vi "Target3.vi"() -> ()   [LabVIEW 2025]
uses:
  <vilib>/Platform/TimedLoop/XDataNode/timing_clust.ctl
  <vilib>/Platform/TimedLoop/XDataNode/nitl_modes.ctl
  <vilib>/Platform/TimedLoop/XDataNode/wakeup.ctl
  <vilib>/eio/utilities/niEioResolveVilibRelativePath.vi
  <vilib>/rvi/interface/RandomDataEmulation/niFpgaRandomDataHandleErrors.vi
  <vilib>/rvi/Emulation/niFpgaSctlEmulationGetInTimedLoop.vi
  <vilib>/rvi/Emulation/niFpgaEmulationReportErrorSimple.vi
  <vilib>/rvi/Emulation/niFpgaGetClockAttributes.vi
  <vilib>/rvi/Emulation/niFpgaCriticalErrorInLSC.vi
  <vilib>/rvi/linearAlgebra/MatrixMultiply/simVIs/SubVI/nifxpla_MatrixMultiply_SimMatrixSizes.vi
  <vilib>/rvi/linearAlgebra/MatrixMultiply/simVIs/SubVI/nifxpla_MatrixMultiply_Sim4WireAdapterVector.vi
  <vilib>/rvi/linearAlgebra/MatrixMultiply/simVIs/SubVI/nifxpla_MatrixMultiply_SimFrameHandShake.vi
  <vilib>/rvi/linearAlgebra/MatrixMultiply/simVIs/SubVI/nifxpla_MatrixMultiply_SimEndlessCounter.vi
  <vilib>/rvi/linearAlgebra/MatrixMultiply/simVIs/SubVI/nifxpla_MatrixMultiply_SimVectorDataBuffer.vi
  <vilib>/rvi/ClientSDK/Core/DevComputerLib/Private/Multiply(dfxp64).vi
  <vilib>/rvi/ClientSDK/Core/DevComputerLib/Private/Dfxp128ToDfxp256.vi
  <vilib>/rvi/ClientSDK/Core/DevComputerLib/Private/Add(dfxp256).vi
  <vilib>/rvi/ClientSDK/Core/DevComputerLib/Private/Subtract(dfxp256).vi
  <vilib>/rvi/ClientSDK/Core/DevComputerLib/Private/ToDfxp64(dfxp256).vi
  <vilib>/rvi/interface/RandomDataEmulation/nirviRandomDataMultiElementFPGAFIFO.vi
  <instcachedir>/0/nirviRandomDataMultiElementFPGAFIFO_BE2FF10D3D6E420AB0291A02835C249E.lvgen/nirviRandomDataMultiElementFPGAFIFO_BE2FF10D3D6E420AB0291A02835C249E_001.vi
  <vilib>/rvi/DataTransferAndStorage/Container/XNode/niFpgaContainer.xnode
  <vilib>/rvi/interface/RandomDataEmulation/nirviRandomDataFpgaReadWriteTemplate.vi
  <vilib>/platform/TimedLoop/XDataNode/XDataNode.xnode
  <vilib>/rvi/linearAlgebra/MatrixMultiply/XNode/nifxpla_MatrixMultiply.xnode
  <vilib>/rvi/linearAlgebra/MatrixMultiply/simVIs/nifxpla_MatrixMultiply_SimTemplateEinEout.vi
  <vilib>/rvi/linearAlgebra/MatrixMultiply/simVIs/nifxpla_MatrixMultiply_SimTemplateEinVout.vi
  <vilib>/rvi/linearAlgebra/MatrixMultiply/simVIs/nifxpla_MatrixMultiply_SimTemplateVinEout.vi
  <vilib>/rvi/linearAlgebra/MatrixMultiply/simVIs/nifxpla_MatrixMultiply_SimTemplateVinVout.vi
  <vilib>/rvi/interface/RandomDataEmulation/nirviRandomDataFpgaMultiElementTemplate.vi
  <vilib>/Platform/TimedLoop/XDataNode/XDNodeRunTimeDep.lvlib
panel:
  out "=0?2":bool
  out "=0?1":bool
  out "ready for b":bool[](array[boolean])
  out "ready for a":bool[](array[boolean])
  out "And 1":bool[](array[boolean])
  out "And 2":bool[](array[boolean])
  out "element 2":fxp<+/-,32,16>
  out "element":fxp<+/-,32,16>
  out "cr":fxp<+/-,32,16>[](array[numeric])
  out "Numeric 2":i32
  out "Array 3":fxp<+/-,32,16>[](array[numeric])
  out "Numeric":i32
  out "appended array 2":fxp<+/-,32,16>[](array[numeric])
  out "appended array":fxp<+/-,32,16>[](array[numeric])
  out "Ready for Input":bool
  out "output valid":bool
  out "operation overflow":bool
  out "Array 4":fxp<+/-,32,16>[](array[numeric])
  out "Array 5":fxp<+/-,32,16>[](array[numeric])
  out "Array 2":bool[](array[boolean])
  out "Array":bool[](array[boolean])
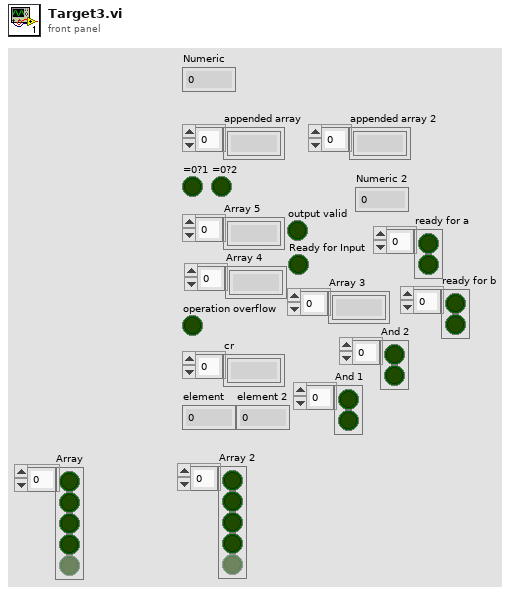
[diagram p1: front panel]
types:
  T1 = typedef "XDNodeRunTimeDep.lvlib/timing_clust.ctl" = cluster{"Expected End [f-1]":u64, "Actual End [f-1]":u64, "Finished Late? [f-1]":bool, "Expected End [i-1]":u64, "Actual End [i-1]":u64, "Finished Late? [i-1]":bool, "Expected Start [i]":u64, "Actual Start [i]":u64, "Expected Start [f]":u64, "Actual Start [f]":u64, "Source Name":string, "Structure Name":string, "Period":i64, "Deadline":i64, "Offset":i64, "Start":i64, "Priority":i32, "Timeout":i32, "Mode":T2, "Wakeup Reason":T3, "Error":errorcluster, "Source Type":string, "Secondary Source Type":string, "Global End Time":u64, "Global Start Time":u64, "Frame Duration":u64, "Iteration Duration":u64, "Assigned CPU":i32, "I/O Scan Engine Mode":u32}
  T2 = typedef "XDNodeRunTimeDep.lvlib/nitl_modes.ctl" = enum32{"No Change", "Process missed periods, maintain original phase", "Discard missed periods, maintain original phase", "Process missed periods, ignore original phase", "Discard missed periods, ignore original phase"}
  T3 = typedef "XDNodeRunTimeDep.lvlib/wakeup.ctl" = enum32{"Normal", "Aborted", "Asynchronous wakeup", "Timing source error", "Timed loop error", "Timeout"}
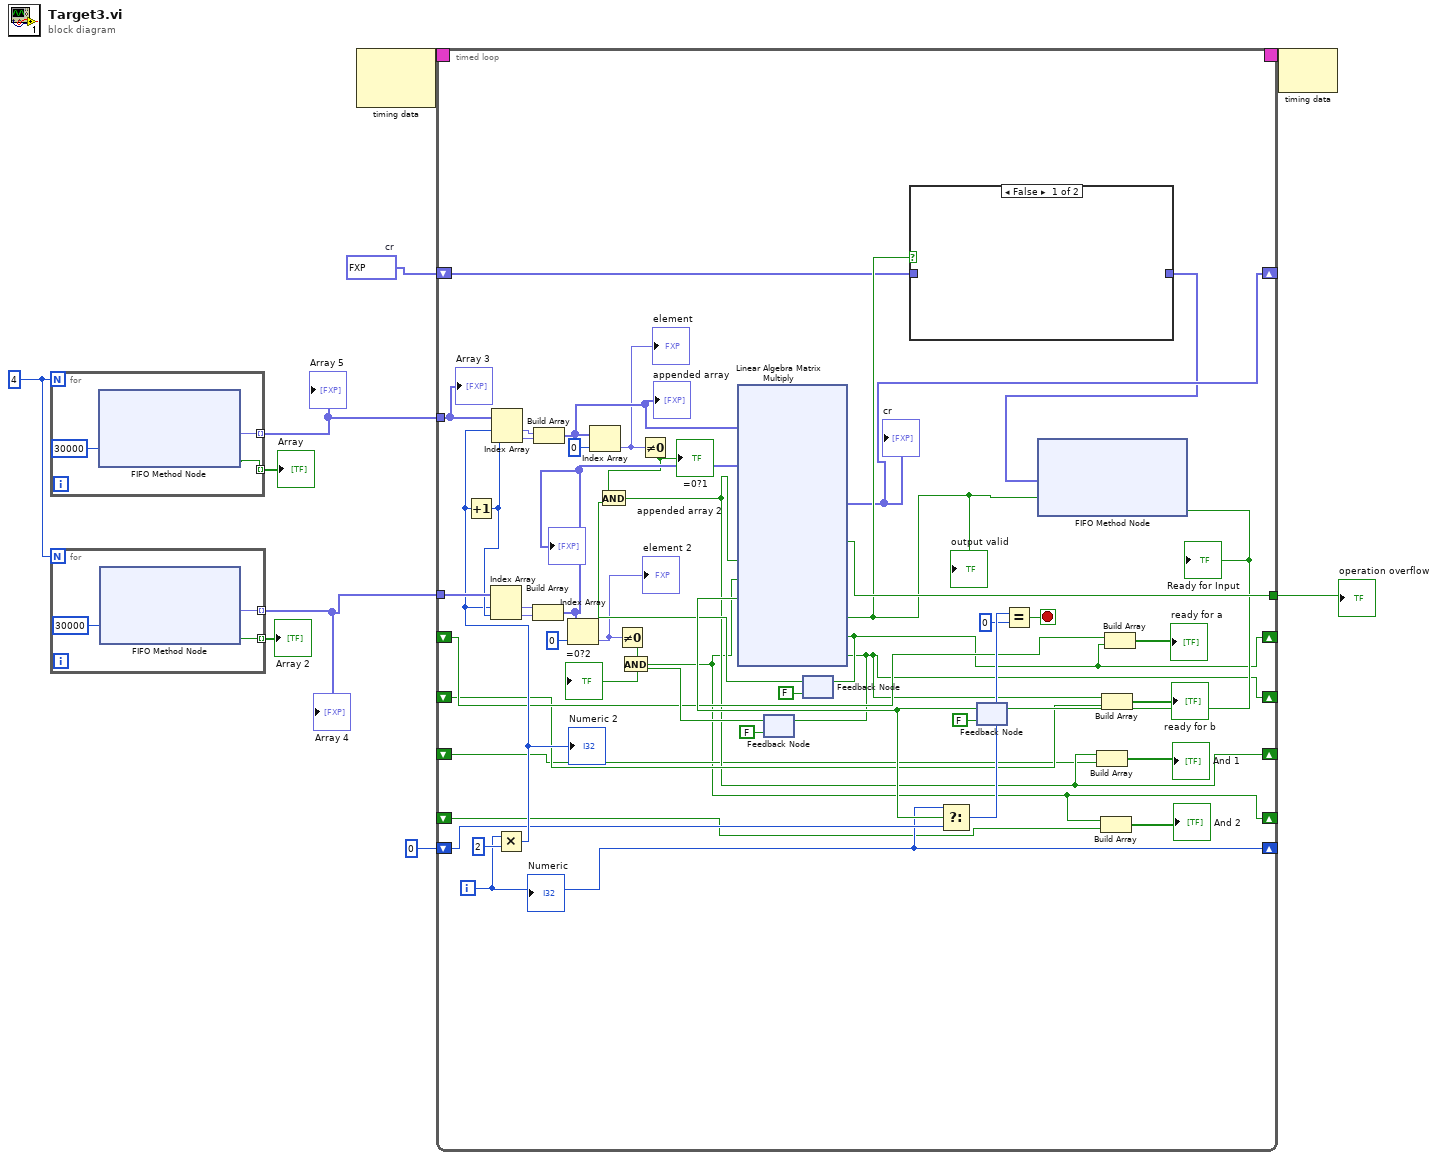
[diagram p0: block diagram]
diagram:
  w1 = fxp<+/-,64,32>[] [0.0, 0.0]  # cr
  w8 = 4
  n1 = for {
    N: w8 -> [_]
    tunnel: [w13] -> w4 mode=indexing
    tunnel: [w11] -> w7 mode=indexing
    n2 = xnode ("FIFO Method Node")("Timeout"=30000) -> ("Element"=w13:fxp<+/-,32,16>, "Timed Out?"=w11:bool)  [unwired: 1 in, 1 out]
  }
  "Array" <- w7
  "Array 5" <- w4
  n3 = for {
    N: w8 -> [_]
    tunnel: [w16] -> w3 mode=indexing
    tunnel: [w14] -> w6 mode=indexing
    n4 = xnode ("FIFO Method Node")("Timeout"=30000) -> ("Element"=w16:fxp<+/-,32,16>, "Timed Out?"=w14:bool)  [unwired: 1 in, 1 out]
  }
  "Array 2" <- w6
  "Array 4" <- w3
  n5 = node-c288() -> (w10:T1)  [unwired: 2 in]
  n6 = timed-loop {
    timing: w10 -> [_]
    timing-out: [_] -> w9
    tunnel: w4 -> [w49]
    tunnel: w3 -> [w60]
    tunnel: [w52] -> w5
    shift-right: [w45] -> _
    shift-left: 0 -> [w46]
    shift-right: [w39] -> _
    shift-left: _ -> [w40]
    shift-right: [w34] -> _
    shift-left: _ -> [w33]
    shift-right: [w32] -> _
    shift-left: _ -> [w31]
    shift-right: [w29] -> _
    shift-left: _ -> [w30]
    shift-right: [w18] -> _
    shift-left: w1 -> [w23]
    i -> [w45]
    stop <- w56 stop-if-true
    n7 = Multiply(x=w45, y=2) -> (x*y=w47:i32)
    "Numeric 2" <- w47
    n8 = Increment(x=w47) -> (x+1=w50:i32)
    n9 = Index Array(array=w60, index #1=w47, index #2=w50) -> (element #1=w61:fxp<+/-,32,16>, element #2=w44:fxp<+/-,32,16>)
    n10 = Index Array(array=w49, index #1=w47, index #2=w50) -> (element #1=w62:fxp<+/-,32,16>, element #2=w22:fxp<+/-,32,16>)
    n11 = Build Array(w61, w44) -> (w26:fxp<+/-,32,16>[])
    "appended array 2" <- w26
    n12 = Build Array(w62, w22) -> (w28:fxp<+/-,32,16>[])
    "appended array" <- w28
    n13 = Index Array(array=w26, index=0) -> (element=w20:fxp<+/-,32,16>)
    "element 2" <- w20
    n14 = Index Array(array=w28, index=0) -> (element=w21:fxp<+/-,32,16>)
    "element" <- w21
    n15 = Not Equal To 0?(x=w20) -> (x != 0?=w43:bool)
    "=0?2" <- w43
    n16 = Not Equal To 0?(x=w21) -> (x != 0?=w19:bool)
    "=0?1" <- w19
    n17 = feedback #1(FALSE ("ready for b")) -> (w42:bool)
    n18 = And(x=w43, y=w42) -> (x .and. y?=w29:bool)
    n19 = feedback #2(FALSE ("ready for a")) -> (w41:bool)
    n20 = And(x=w19, y=w41) -> (x .and. y?=w32:bool)
    n21 = feedback #3(FALSE ("Ready for Input")) -> (w57:bool)
    n22 = xnode ("Linear Algebra Matrix Multiply")("ar"=w28, "br"=w26, "a valid"=w32, "b valid"=w29, "ready for output (T)"=w57) -> ("cr"=w18:fxp<+/-,64,32>[], "operation overflow"=w52:bool, "output valid"=w24:bool, "ready for a"=w39:bool, "ready for b"=w34:bool)  [unwired: 2 in, 1 out]
    "output valid" <- w24
    "cr" <- w18
    n23 = feedback-in #1(w34) -> ()
    n24 = feedback-in #2(w39) -> ()
    n25 = case shown="False" w24 {
      tunnel: w23 -> [_ w63]
      tunnel: [_ w63] -> w17
      frame False {
      }
      frame True {
      }
    }
    n26 = Select(t=w45, s=w57, f=w46) -> (s? t:f=w55:i32)
    n27 = Equal?(x=w55, y=0) -> (x = y?=w56:bool)
    n28 = xnode ("FIFO Method Node")("Element"=w17, "Input Valid"=w24) -> ("Ready for Input"=w51:bool)  [unwired: 1 in, 1 out]
    "Ready for Input" <- w51
    n29 = feedback-in #3(w51) -> ()
    n30 = Build Array(w32, w31) -> (→"And 1":bool[])
    n31 = Build Array(w29, w30) -> (→"And 2":bool[])
    n32 = Build Array(w34, w33) -> (→"ready for b":bool[])
    n33 = Build Array(w40, w39) -> (→"ready for a":bool[])
    "Numeric" <- w45
    "Array 3" <- w49
  }
  "operation overflow" <- w5
  n34 = node-c288(w9) -> ()  [unwired: 1 out]
